vi "prop_cursor_main.vi"() -> ()   [LabVIEW 2020, in "3DPC_SurfacePlot.xctl"]
uses:
  <vilib>/Native 3D Graph/xcontrol/3DPC_SurfacePlot.xctl
  <vilib>/Native 3D Graph/typedefs/prop_cursor_all_array.ctl
  <vilib>/Native 3D Graph/typedefs/prop_cursor_point.ctl
  <vilib>/Native 3D Graph/typedefs/prop_cursor_position.ctl
  <vilib>/Native 3D Graph/typedefs/prop_cursor_line.ctl
  <vilib>/Native 3D Graph/typedefs/prop_cursor_plane.ctl
  <vilib>/Native 3D Graph/typedefs/prop_cursor_text.ctl
  <vilib>/Utility/miscctls.llb/LVPointTypeDef.ctl
panel:
  in  "Cursorname":string="Cursor"
  in  "Plot IDs":i32[](array[numeric])
  in  "done":refnum<user-event>
  in  "quit":refnum<user-event>
  out "Cursor Properties Array Out":T1
  in  "Cursor Properties Array In":T1
  in  "Cursor Enable":bool
  in  "Cursor Visible":bool
  in  "Delete Cursor":bool
  in  "Add Cursor":bool
  in  "Cursor List":i32(listbox)
  in  "Tab Plot Prop":T7(tab)
  in  "Position X":dbl caption="X"
  in  "Position Y":dbl caption="Y"
  in  "Position Z":dbl caption="Z"
  in  "Position Snap To":u16(ring) caption="Snap to" items=["Fixed", "Nearest Plot", "Snap to Plot"]
  in  "Polsition Pick Plot":u16(ring) caption="Plot"
  in  "Point Color":u32(colorbox) caption="Color"
  in  "Point Size":dbl caption="Size"
  in  "Point Visible":bool
  in  "Line Color":u32(colorbox) caption="Color"
  in  "Line Width":dbl caption="Width"
  in  "Line Visible":bool
  in  "Plane Opacity":dbl caption="Opacity"
  in  "Plane Color":u32(colorbox) caption="Color"
  in  "Plane XY":bool
  in  "Plane XZ":bool
  in  "Plane YZ":bool
  in  "Text Color":u32(colorbox)
  in  "Text Back Color":u32(colorbox) caption="Back Color"
  in  "Text Font Size":i32 caption="Font Size"
  in  "Text Opacity":dbl caption="Opacity"
  in  "Text Show Position":bool caption="Show Position"
  in  "Text Show Name":bool
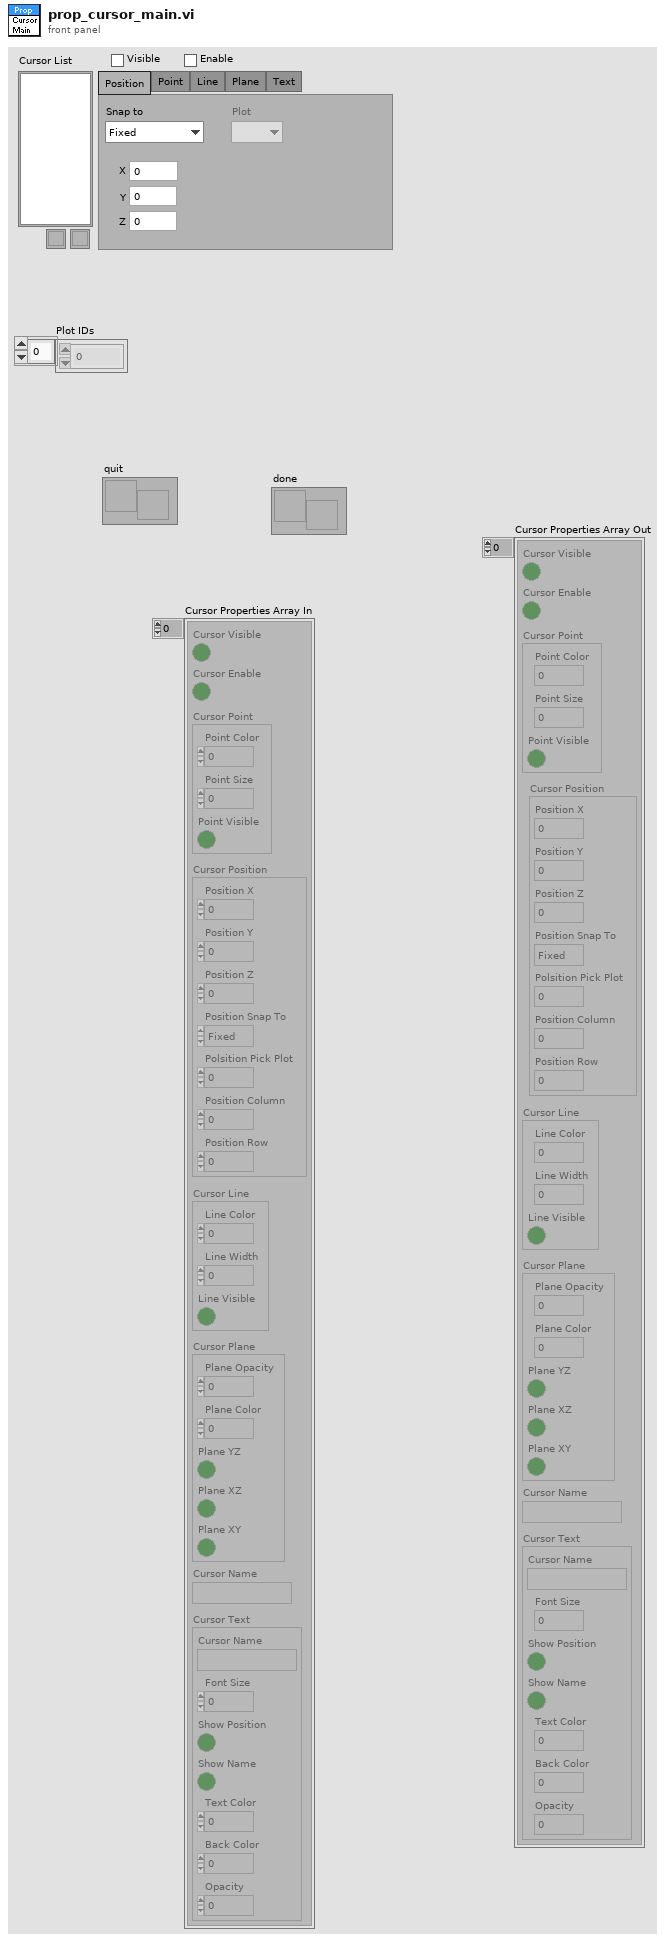
[diagram p1: front panel]
types:
  T1 = typedef "3DPC_SurfacePlot.xctl/prop_cursor_all_array.ctl" = cluster{"Cursor Visible":bool, "Cursor Enable":bool, "Cursor Point":T2, "Cursor Position":T3, "Cursor Line":T4, "Cursor Plane":T5, "Cursor Name":string, "Cursor Text":T6}[]
  T2 = typedef "3DPC_SurfacePlot.xctl/prop_cursor_point.ctl" = cluster{"Point Color":u32, "Point Size":dbl, "Point Visible":bool}
  T3 = typedef "3DPC_SurfacePlot.xctl/prop_cursor_position.ctl" = cluster{"Position X":dbl, "Position Y":dbl, "Position Z":dbl, "Position Snap To":enum16{"Fixed", "Nearest Plot", "Snap to Plot"}, "Polsition Pick Plot":u16, "Position Column":i32, "Position Row":i32}
  T4 = typedef "3DPC_SurfacePlot.xctl/prop_cursor_line.ctl" = cluster{"Line Color":u32, "Line Width":dbl, "Line Visible":bool}
  T5 = typedef "3DPC_SurfacePlot.xctl/prop_cursor_plane.ctl" = cluster{"Plane Opacity":dbl, "Plane Color":u32, "Plane YZ":bool, "Plane XZ":bool, "Plane XY":bool}
  T6 = typedef "3DPC_SurfacePlot.xctl/prop_cursor_text.ctl" = cluster{"Cursor Name":string, "Font Size":i32, "Show Position":bool, "Show Name":bool, "Text Color":u32, "Back Color":u32, "Opacity":dbl}
  T7 = enum32{"Position", "Point", "Line", "Plane", "Text"}
  T8 = typedef "LVPointTypeDef.ctl" = cluster{"Horizontal":i16, "Vertical":i16}
  T9 = cluster{"Cursor Visible":bool, "Cursor Enable":bool, "Cursor Point":T2, "Cursor Position":T3, "Cursor Line":T4, "Cursor Plane":T5, "Cursor Name":string, "Cursor Text":T6}
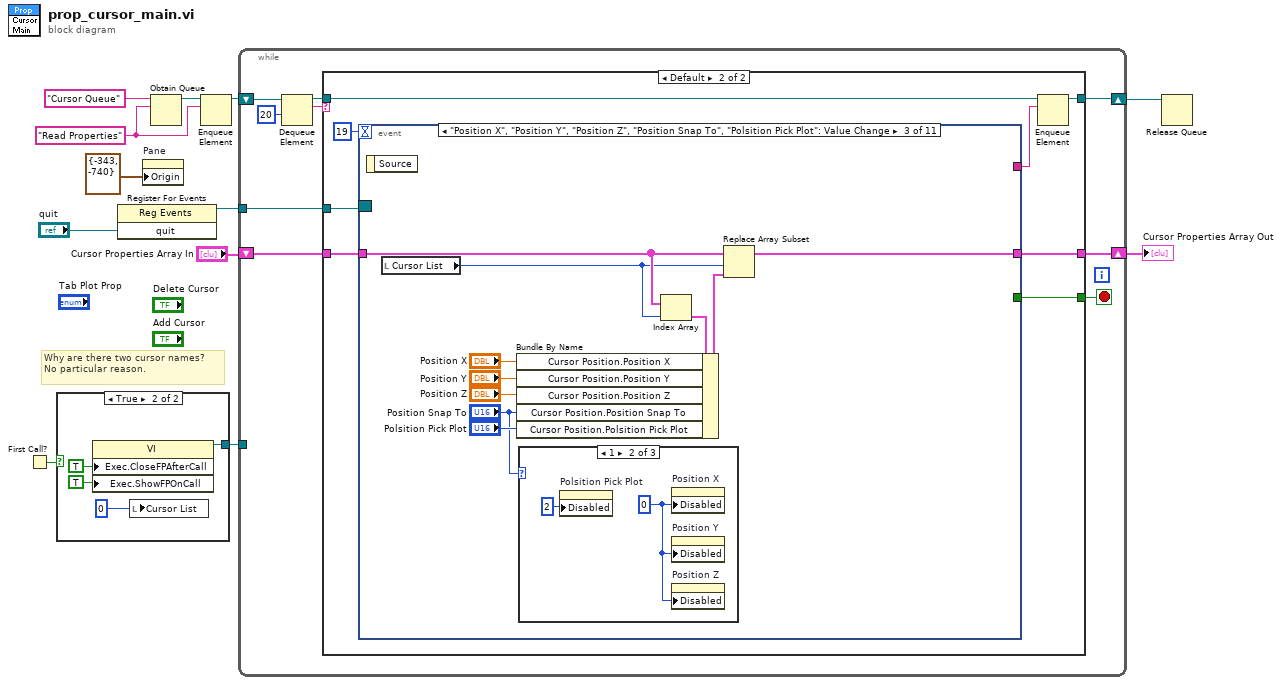
[diagram p0: block diagram]
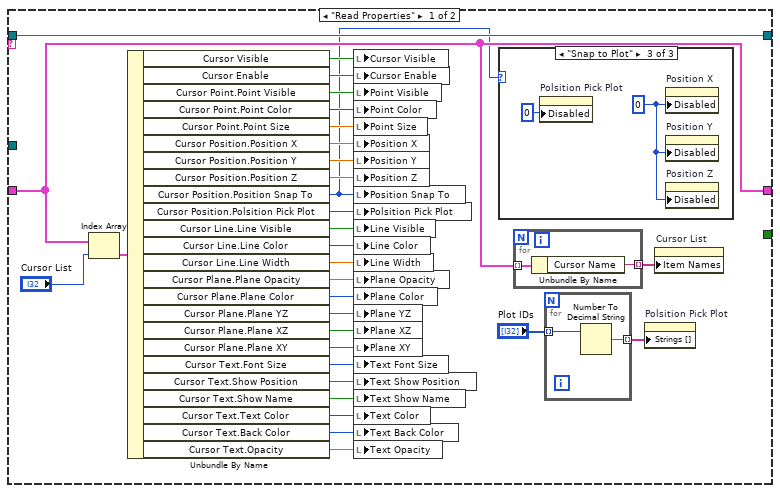
[diagram p3: hidden frame]
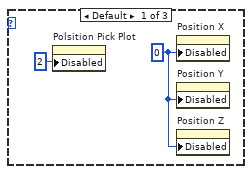
[diagram p4: hidden frame]
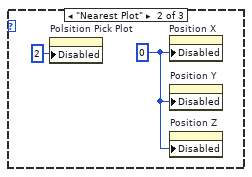
[diagram p5: hidden frame]
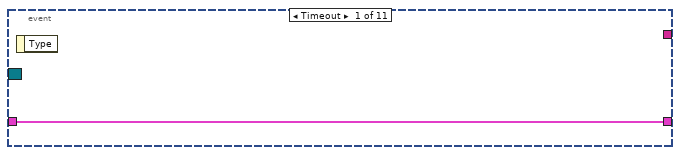
[diagram p6: hidden frame]
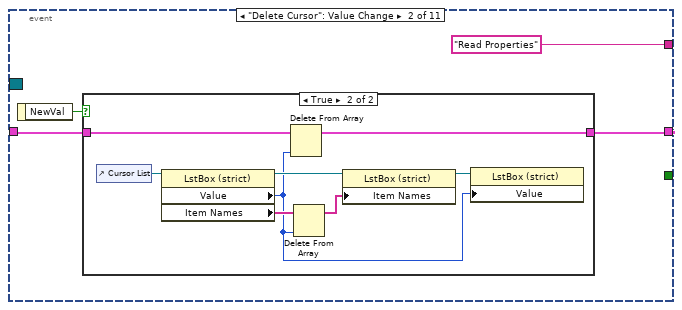
[diagram p7: hidden frame]
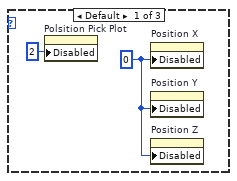
[diagram p9: hidden frame]
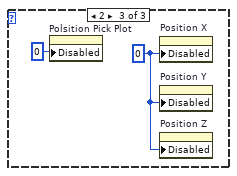
[diagram p10: hidden frame]
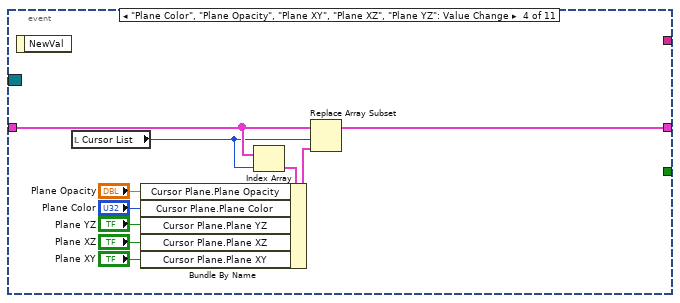
[diagram p11: hidden frame]
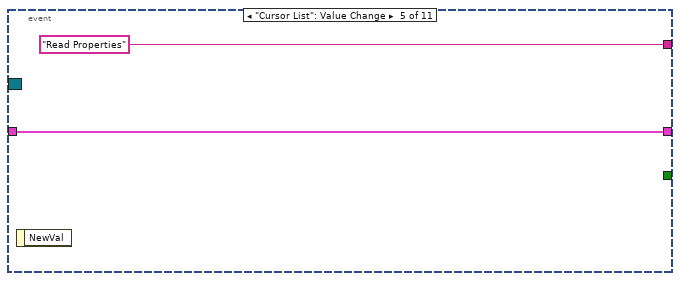
[diagram p12: hidden frame]
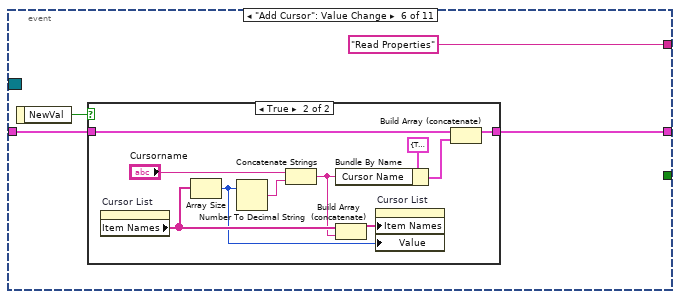
[diagram p13: hidden frame]
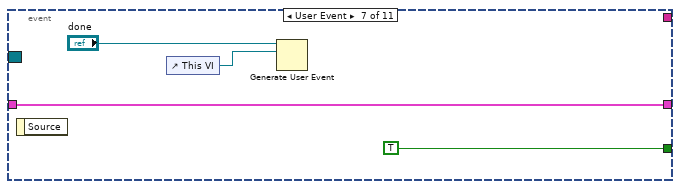
[diagram p15: hidden frame]
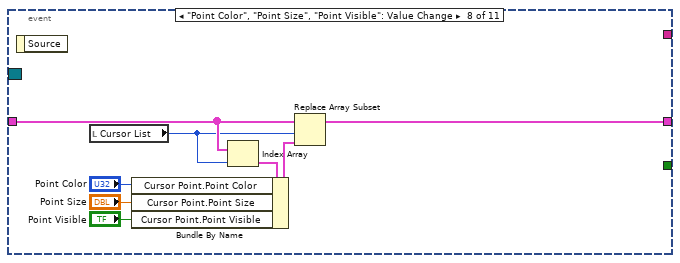
[diagram p16: hidden frame]
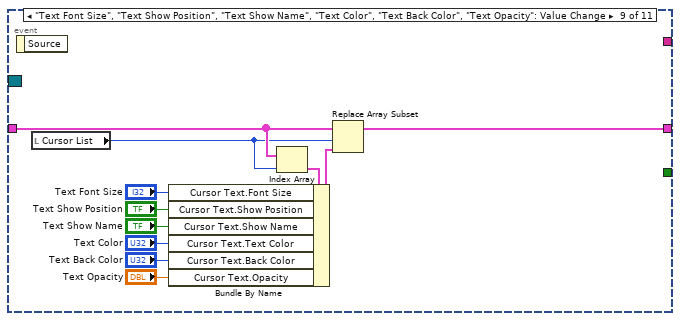
[diagram p17: hidden frame]
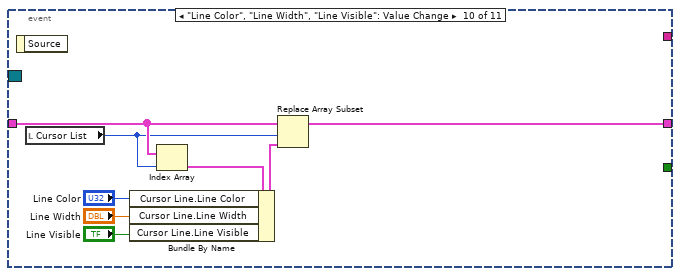
[diagram p18: hidden frame]
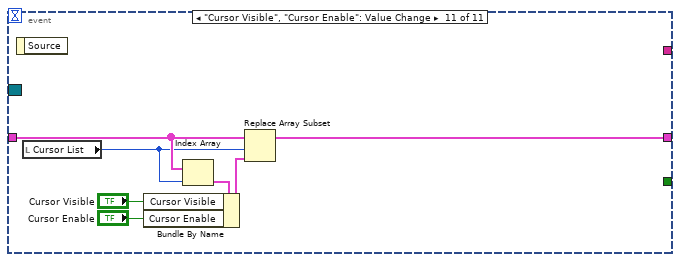
[diagram p19: hidden frame]
diagram:
  w10 = "Read Properties"
  # "Why are there two cursor names?  No particular reason."
  n1 = First Call?() -> (First Call?: T/F=w1:bool)
  n2 = case shown="True" w1 {
    tunnel: [_ w14] -> w7
    frame False {
    }
    frame True {
      n3 = property class="VI"("Exec.CloseFPAfterCall"=TRUE ("Execution:Close After Call"), "Exec.ShowFPOnCall"=TRUE ("Execution:Show Front Panel On Call")) -> (reference out=w14:refnum<vi>)  [unwired: 2 in, 1 out]
      n4 = local write "Cursor List"(0 ("Cursors:")) -> ()
    }
  }
  n5 = register-events("quit") -> (reference out=w3:refnum<event-registration>)  [unwired: 2 in, 1 out]
  n6 = property on="Pane" class="Pane"("Origin"=T8 {"Horizontal"=-343, "Vertical"=-740}) -> ()  [unwired: 2 in, 2 out]
  n7 = Obtain Queue(name (unnamed)="Cursor Queue", element data type=w10) -> (queue out=w11:refnum<queue>)  [unwired: 3 in, 2 out]
  n8 = Enqueue Element(queue=w11, element=w10) -> (queue out=w9:refnum<queue>)  [unwired: 1 in, 3 out]
  n9 = while {
    shift-right: [w24] -> w5
    shift-left: "Cursor Properties Array In" -> [w25]
    shift-right: [w19] -> w8
    shift-left: w9 -> [w22]
    tunnel: w7 -> [_]
    tunnel: w3 -> [w18]
    stop <- w17 stop-if-true
    n10 = Dequeue Element(queue=w22, timeout in ms (-1)=20) -> (queue out=w20:refnum<queue>, element=w21:string)  [unwired: 1 in, 2 out]
    n11 = case shown="Default" w21 {
      tunnel: w25 -> [w37 w71]
      tunnel: [w37 w70] -> w24
      tunnel: w20 -> [w56 w74]
      tunnel: [_ w67] -> w17
      tunnel: [w56 w73] -> w19
      tunnel: w18 -> [_ w68]
      frame "Read Properties" {
        n12 = Index Array(array=w37, index="Cursor List") -> (element=w55:T9)
        n13 = Unbundle By Name(w55) -> ("Cursor Visible"=w54:bool, "Cursor Enable"=w53:bool, "Cursor Point.Point Visible"=w39:bool, "Cursor Point.Point Color"=w52:u32, "Cursor Point.Point Size"=w51:dbl, "Cursor Position.Position X"=w50:dbl, "Cursor Position.Position Y"=w49:dbl, "Cursor Position.Position Z"=w48:dbl, "Cursor Position.Position Snap To"=w26:enum16{"Fixed", "Nearest Plot", "Snap to Plot"}, "Cursor Position.Polsition Pick Plot"=w47:u16, "Cursor Line.Line Visible"=w38:bool, "Cursor Line.Line Color"=w46:u32, "Cursor Line.Line Width"=w45:dbl, "Cursor Plane.Plane Opacity"=w44:dbl, "Cursor Plane.Plane Color"=w43:u32, "Cursor Plane.Plane YZ"=w42:bool, "Cursor Plane.Plane XZ"=w41:bool, "Cursor Plane.Plane XY"=w40:bool, "Cursor Text.Font Size"=w36:i32, "Cursor Text.Show Position"=w35:bool, "Cursor Text.Show Name"=w34:bool, "Cursor Text.Text Color"=w33:u32, "Cursor Text.Back Color"=w32:u32, "Cursor Text.Opacity"=w31:dbl)
        n14 = local write "Cursor Visible"(w54) -> ()
        n15 = local write "Cursor Enable"(w53) -> ()
        n16 = local write "Point Visible"(w39) -> ()
        n17 = local write "Point Color"(w52) -> ()
        n18 = local write "Point Size"(w51) -> ()
        n19 = local write "Position X"(w50) -> ()
        n20 = local write "Position Y"(w49) -> ()
        n21 = local write "Position Z"(w48) -> ()
        n22 = local write "Position Snap To"(w26) -> ()
        n23 = local write "Polsition Pick Plot"(w47) -> ()
        n24 = local write "Line Visible"(w38) -> ()
        n25 = local write "Line Color"(w46) -> ()
        n26 = local write "Line Width"(w45) -> ()
        n27 = local write "Plane Opacity"(w44) -> ()
        n28 = local write "Plane Color"(w43) -> ()
        n29 = local write "Plane YZ"(w42) -> ()
        n30 = local write "Plane XZ"(w41) -> ()
        n31 = local write "Plane XY"(w40) -> ()
        n32 = local write "Text Font Size"(w36) -> ()
        n33 = local write "Text Show Position"(w35) -> ()
        n34 = local write "Text Show Name"(w34) -> ()
        n35 = local write "Text Color"(w33) -> ()
        n36 = local write "Text Back Color"(w32) -> ()
        n37 = local write "Text Opacity"(w31) -> ()
        n38 = case shown="\"Snap to Plot\"" w26 {
          frame Default {
            w57 = u8 0 ("Disabled")
            n39 = property on="Polsition Pick Plot" class="Ring (strict)"("Disabled"=u8 2) -> ()  [unwired: 2 in, 2 out]
            n40 = property on="Position X" class="DigNum (strict)"("Disabled"=w57) -> ()  [unwired: 2 in, 2 out]
            n41 = property on="Position Y" class="DigNum (strict)"("Disabled"=w57) -> ()  [unwired: 2 in, 2 out]
            n42 = property on="Position Z" class="DigNum (strict)"("Disabled"=w57) -> ()  [unwired: 2 in, 2 out]
          }
          frame "Nearest Plot" {
            w59 = u8 0 ("Disabled")
            n43 = property on="Polsition Pick Plot" class="Ring (strict)"("Disabled"=u8 2) -> ()  [unwired: 2 in, 2 out]
            n44 = property on="Position X" class="DigNum (strict)"("Disabled"=w59) -> ()  [unwired: 2 in, 2 out]
            n45 = property on="Position Y" class="DigNum (strict)"("Disabled"=w59) -> ()  [unwired: 2 in, 2 out]
            n46 = property on="Position Z" class="DigNum (strict)"("Disabled"=w59) -> ()  [unwired: 2 in, 2 out]
          }
          frame "Snap to Plot" {
            w61 = u8 0 ("Disabled")
            n47 = property on="Polsition Pick Plot" class="Ring (strict)"("Disabled"=u8 0) -> ()  [unwired: 2 in, 2 out]
            n48 = property on="Position X" class="DigNum (strict)"("Disabled"=w61) -> ()  [unwired: 2 in, 2 out]
            n49 = property on="Position Y" class="DigNum (strict)"("Disabled"=w61) -> ()  [unwired: 2 in, 2 out]
            n50 = property on="Position Z" class="DigNum (strict)"("Disabled"=w61) -> ()  [unwired: 2 in, 2 out]
          }
        }
        n51 = for {
          tunnel: w37 -> [w66] mode=indexing
          tunnel: [w65] -> w28 mode=indexing
          n52 = Unbundle By Name(w66) -> ("Cursor Name"=w65:string)
        }
        n53 = for {
          tunnel: "Plot IDs" -> [w64] mode=indexing
          tunnel: [w63] -> w29 mode=indexing
          n54 = Number To Decimal String(number=w64) -> (decimal integer string=w63:string)  [unwired: 1 out]
        }
        n55 = property on="Polsition Pick Plot" class="Ring (strict)"("Strings []"=w29) -> ()  [unwired: 2 in, 2 out]
        n56 = property on="Cursor List" class="LstBox (strict)"("Item Names"=w28) -> ()  [unwired: 2 in, 2 out]
      }
      frame Default {
        n57 = event shown="[2] \"Position X\", \"Position Y\", \"Position Z\", \"Position Snap To\", \"Polsition Pick Plot\": Value Change" {
          selector: w68 -> [_ _ _ _ _ _ _ _ _ _ _]
          dyn-events: _ -> [_ _ _ _ _ _ _ _ _ _ _]
          timeout: 19 -> [_ _ _ _ _ _ _ _ _ _ _]
          tunnel: [_ "Read Properties" ("element") _ _ "Read Properties" ("element") "Read Properties" ("element") _ _ _ _ _] -> w72
          tunnel: w71 -> [w75 w78 w91 w112 w115 w119 w132 w140 w154 w160 w167]
          tunnel: [w75 w77 w96 w111 w115 w118 w132 w141 w153 w159 w166] -> w70
          tunnel: [_ _ _ _ _ _ TRUE _ _ _ _] -> w67
          event Timeout {
            n58 = event-data() -> ()  [unwired: 2 out]
          }
          event "Delete Cursor": Value Change {
            n59 = event-data() -> ("NewVal"=w79:bool)  [unwired: 1 out]
            n60 = case shown="True" w79 {
              tunnel: w78 -> [w80 w88]
              tunnel: [w80 w87] -> w77
              frame False {
              }
              frame True {
                n61 = control-ref of="Cursor List"() -> (w84:refnum<vi>)
                n62 = property on="Property Node" class="LstBox (strict)"(reference=w84) -> (reference out=w83:refnum<vi>, "Value"=w81:i32, "Item Names"=w86:string[])  [unwired: 1 in, 1 out]
                n63 = Delete From Array(array=w88, index=w81) -> (array with subset deleted=w87:T1)  [unwired: 1 in, 1 out]
                n64 = Delete From Array(array=w86, index=w81) -> (array with subset deleted=w85:string[])  [unwired: 1 in, 1 out]
                n65 = property on="Property Node" class="LstBox (strict)"(reference=w83, "Item Names"=w85) -> (reference out=w82:refnum<vi>)  [unwired: 1 in, 1 out]
                n66 = property class="LstBox (strict)"(reference=w82, "Value"=w81) -> ()  [unwired: 1 in, 2 out]
              }
            }
          }
          event "Position X", "Position Y", "Position Z", "Position Snap To", "Polsition Pick Plot": Value Change {
            n67 = event-data() -> ()  [unwired: 2 out]
            n68 = local read "Cursor List"() -> (w89:i32)
            n69 = case shown="1" "Position Snap To" {
              frame Default {
                w99 = u8 0 ("Disabled")
                n70 = property on="Polsition Pick Plot" class="Ring (strict)"("Disabled"=u8 2) -> ()  [unwired: 2 in, 2 out]
                n71 = property on="Position X" class="DigNum (strict)"("Disabled"=w99) -> ()  [unwired: 2 in, 2 out]
                n72 = property on="Position Y" class="DigNum (strict)"("Disabled"=w99) -> ()  [unwired: 2 in, 2 out]
                n73 = property on="Position Z" class="DigNum (strict)"("Disabled"=w99) -> ()  [unwired: 2 in, 2 out]
              }
              frame 1 {
                w101 = u8 0 ("Disabled")
                n74 = property on="Polsition Pick Plot" class="Ring (strict)"("Disabled"=u8 2) -> ()  [unwired: 2 in, 2 out]
                n75 = property on="Position X" class="DigNum (strict)"("Disabled"=w101) -> ()  [unwired: 2 in, 2 out]
                n76 = property on="Position Y" class="DigNum (strict)"("Disabled"=w101) -> ()  [unwired: 2 in, 2 out]
                n77 = property on="Position Z" class="DigNum (strict)"("Disabled"=w101) -> ()  [unwired: 2 in, 2 out]
              }
              frame 2 {
                w103 = u8 0 ("Disabled")
                n78 = property on="Polsition Pick Plot" class="Ring (strict)"("Disabled"=u8 0) -> ()  [unwired: 2 in, 2 out]
                n79 = property on="Position X" class="DigNum (strict)"("Disabled"=w103) -> ()  [unwired: 2 in, 2 out]
                n80 = property on="Position Y" class="DigNum (strict)"("Disabled"=w103) -> ()  [unwired: 2 in, 2 out]
                n81 = property on="Position Z" class="DigNum (strict)"("Disabled"=w103) -> ()  [unwired: 2 in, 2 out]
              }
            }
            n82 = Index Array(array=w91, index=w89) -> (element=w98:T9)
            n83 = Bundle By Name(cluster=w98, "Cursor Position.Position X"="Position X", "Cursor Position.Position Y"="Position Y", "Cursor Position.Position Z"="Position Z", "Cursor Position.Position Snap To"="Position Snap To", "Cursor Position.Polsition Pick Plot"="Polsition Pick Plot") -> (w97:T9)
            n84 = Replace Array Subset(array=w91, new element=w97, index=w89) -> (w96:T1)
          }
          event "Plane Color", "Plane Opacity", "Plane XY", "Plane XZ", "Plane YZ": Value Change {
            n85 = event-data() -> ()  [unwired: 2 out]
            n86 = local read "Cursor List"() -> (w105:i32)
            n87 = Index Array(array=w112, index=w105) -> (element=w114:T9)
            n88 = Bundle By Name(cluster=w114, "Cursor Plane.Plane Opacity"="Plane Opacity", "Cursor Plane.Plane Color"="Plane Color", "Cursor Plane.Plane YZ"="Plane YZ", "Cursor Plane.Plane XZ"="Plane XZ", "Cursor Plane.Plane XY"="Plane XY") -> (w113:T9)
            n89 = Replace Array Subset(array=w112, new element=w113, index=w105) -> (w111:T1)
          }
          event "Cursor List": Value Change {
            n90 = event-data() -> ()  [unwired: 2 out]
          }
          event "Add Cursor": Value Change {
            n91 = event-data() -> ("NewVal"=w120:bool)  [unwired: 1 out]
            n92 = case shown="True" w120 {
              tunnel: w119 -> [w121 w131]
              tunnel: [w121 w130] -> w118
              frame False {
              }
              frame True {
                n93 = property on="Cursor List" class="LstBox (strict)"() -> ("Item Names"=w128:string[])  [unwired: 2 in, 2 out]
                n94 = Array Size(array=w128) -> (size(s)=w124:i32)
                n95 = Number To Decimal String(number=w124) -> (decimal integer string=w126:string)  [unwired: 1 out]
                n96 = Concatenate Strings("Cursorname", w126) -> (w125:string)
                n97 = Bundle By Name(cluster=T9 {"Cursor Visible"=TRUE, "Cursor Enable"=TRUE, "Cursor Point"={"Point Color"=0, "Point Size"=3.0, "Point Visible"=TRUE}, "Cursor Position"={"Position X"=0.0, "Position Y"=0.0, "Position Z"=0.0, "Position Snap To"=enum."Fixed", "Polsition Pick Plot"=0, "Position Column"=0, "Position Row"=0}, "Cursor Line"={"Line Color"=0, "Line Width"=2.0, "Line Visible"=FALSE}, "Cursor Plane"={"Plane Opacity"=0.5, "Plane Color"=0, "Plane YZ"=FALSE, "Plane XZ"=FALSE, "Plane XY"=FALSE}, "Cursor Name"="", "Cursor Text"={"Cursor Name"="", "Font Size"=8, "Show Position"=FALSE, "Show Name"=FALSE, "Text Color"=0, "Back Color"=0, "Opacity"=0.5}} ("Cursor Properties"), "Cursor Name"=w125) -> (w123:T9)
                n98 = Build Array (concatenate)(w128, w125) -> (w129:string[])
                n99 = property on="Cursor List" class="LstBox (strict)"("Item Names"=w129, "Value"=w124) -> ()  [unwired: 2 in, 2 out]
                n100 = Build Array (concatenate)(w131, w123) -> (w130:T1)
              }
            }
          }
          event User Event {
            n101 = event-data() -> ()  [unwired: 2 out]
            n102 = control-ref of="This VI"() -> (w134:refnum<vi>)
            n103 = Generate User Event(user event="done", event data cluster=w134) -> ()  [unwired: 2 in, 2 out]
          }
          event "Point Color", "Point Size", "Point Visible": Value Change {
            n104 = event-data() -> ()  [unwired: 2 out]
            n105 = local read "Cursor List"() -> (w136:i32)
            n106 = Index Array(array=w140, index=w136) -> (element=w143:T9)
            n107 = Bundle By Name(cluster=w143, "Cursor Point.Point Color"="Point Color", "Cursor Point.Point Size"="Point Size", "Cursor Point.Point Visible"="Point Visible") -> (w142:T9)
            n108 = Replace Array Subset(array=w140, new element=w142, index=w136) -> (w141:T1)
          }
          event "Text Font Size", "Text Show Position", "Text Show Name", "Text Color", "Text Back Color", "Text Opacity": Value Change {
            n109 = event-data() -> ()  [unwired: 2 out]
            n110 = local read "Cursor List"() -> (w144:i32)
            n111 = Index Array(array=w154, index=w144) -> (element=w152:T9)
            n112 = Bundle By Name(cluster=w152, "Cursor Text.Font Size"="Text Font Size", "Cursor Text.Show Position"="Text Show Position", "Cursor Text.Show Name"="Text Show Name", "Cursor Text.Text Color"="Text Color", "Cursor Text.Back Color"="Text Back Color", "Cursor Text.Opacity"="Text Opacity") -> (w145:T9)
            n113 = Replace Array Subset(array=w154, new element=w145, index=w144) -> (w153:T1)
          }
          event "Line Color", "Line Width", "Line Visible": Value Change {
            n114 = event-data() -> ()  [unwired: 2 out]
            n115 = local read "Cursor List"() -> (w155:i32)
            n116 = Index Array(array=w160, index=w155) -> (element=w162:T9)
            n117 = Bundle By Name(cluster=w162, "Cursor Line.Line Color"="Line Color", "Cursor Line.Line Width"="Line Width", "Cursor Line.Line Visible"="Line Visible") -> (w161:T9)
            n118 = Replace Array Subset(array=w160, new element=w161, index=w155) -> (w159:T1)
          }
          event "Cursor Visible", "Cursor Enable": Value Change {
            n119 = event-data() -> ()  [unwired: 2 out]
            n120 = local read "Cursor List"() -> (w163:i32)
            n121 = Index Array(array=w167, index=w163) -> (element=w169:T9)
            n122 = Bundle By Name(cluster=w169, "Cursor Visible"="Cursor Visible", "Cursor Enable"="Cursor Enable") -> (w168:T9)
            n123 = Replace Array Subset(array=w167, new element=w168, index=w163) -> (w166:T1)
          }
        }
        n124 = Enqueue Element(queue=w74, element=w72) -> (queue out=w73:refnum<queue>)  [unwired: 1 in, 3 out]
      }
    }
  }
  "Cursor Properties Array Out" <- w5
  n125 = Release Queue(queue=w8) -> ()  [unwired: 1 in, 4 out]
